vi "getMode.vi"(8 "error in (no error)":errorcluster, 11 "Electrometer in":refnum<class "Electrometer.lvclass">) -> (0 "error out":errorcluster, 2 "Mode":string, 3 "Electrometer out":refnum<class "Electrometer.lvclass">)   [LabVIEW 2016, in "Electrometer.lvclass"]
uses:
  Electrometer.lvclass
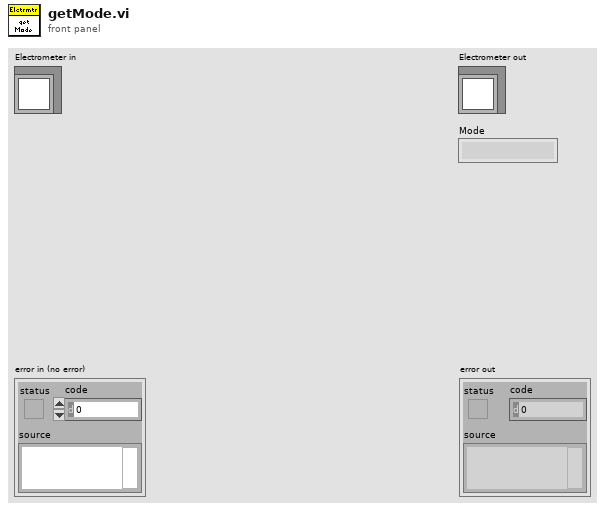
[diagram p1: front panel]
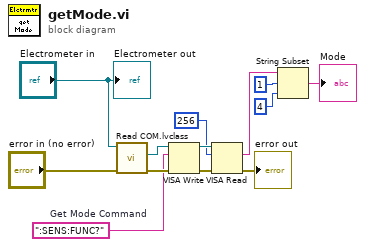
[diagram p0: block diagram]
diagram:
  w11 = ":SENS:FUNC?"  # Get Mode Command
  n1 = call "Read COM.lvclass.vi"("error in (no error)"="error in (no error)", "Electrometer in"="Electrometer in") -> ("error out"=w12:errorcluster, "VISA"=w13:refnum<visa-resource-name>)  [unwired: 7 in, 1 out]
  n2 = VISA Write(VISA resource name=w13, write buffer=w11, error in (no error)=w12) -> (VISA resource name out=w10:refnum<visa-resource-name>, error out=w8:errorcluster)  [unwired: 1 out]
  n3 = VISA Read(VISA resource name=w10, byte count=u32 256, error in (no error)=w8) -> (read buffer=w5:string, error out=→"error out":errorcluster)  [unwired: 2 out]
  n4 = String Subset(string=w5, offset (0)=1, length (rest)=4 ("length (rest)")) -> (substring=→"Mode":string)
  "Electrometer out" <- "Electrometer in"
